vi "Initialize TreeBrowserWF.vi"(7 "guids":string[](array[string])=["4b95dee7-8d64-48ce-932c-f5fdd14e4d4c", "94e87467-031b-484c-a85e-bcbac581524d"], 8 "error in (no error)":errorcluster, 9 "Input Channels":cluster{"Node ID":u64}[](array[cluster]), 10 "Node Pointer":T1, 11 "TreeBrowserRef":refnum<k24>) -> (0 "error out":errorcluster, 2 "Channels":variant, 3 "TreeBrowserRef 2":refnum<k24>)   [LabVIEW 2023, in "Protection and Counter Support System Explorer.lvlib"]
uses:
  Protection and Counter Support System Explorer.lvlib
  <vilib>/NI VeriStand/Custom Device API/Custom Device Pointer.ctl
  NationalInstruments.VeriStand.SystemStorage
  NationalInstruments.VeriStand.SystemStorageUI
  NationalInstruments.VeriStand
  <vilib>/NI VeriStand/Custom Device API/Custom Device API.lvlib
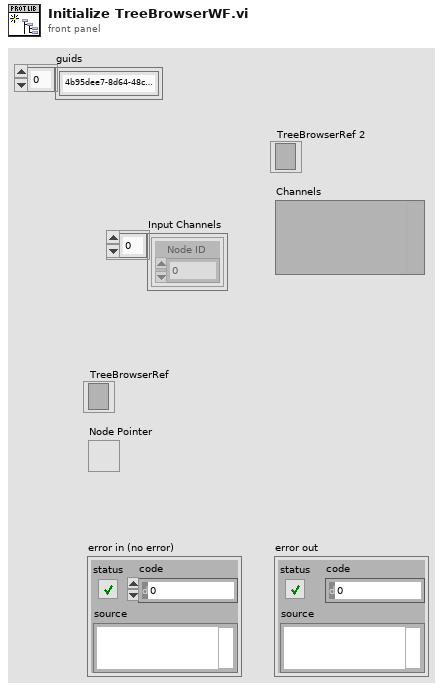
[diagram p1: front panel]
types:
  T1 = typedef "Custom Device API.lvlib/Custom Device Pointer.ctl" = refnum<k24>
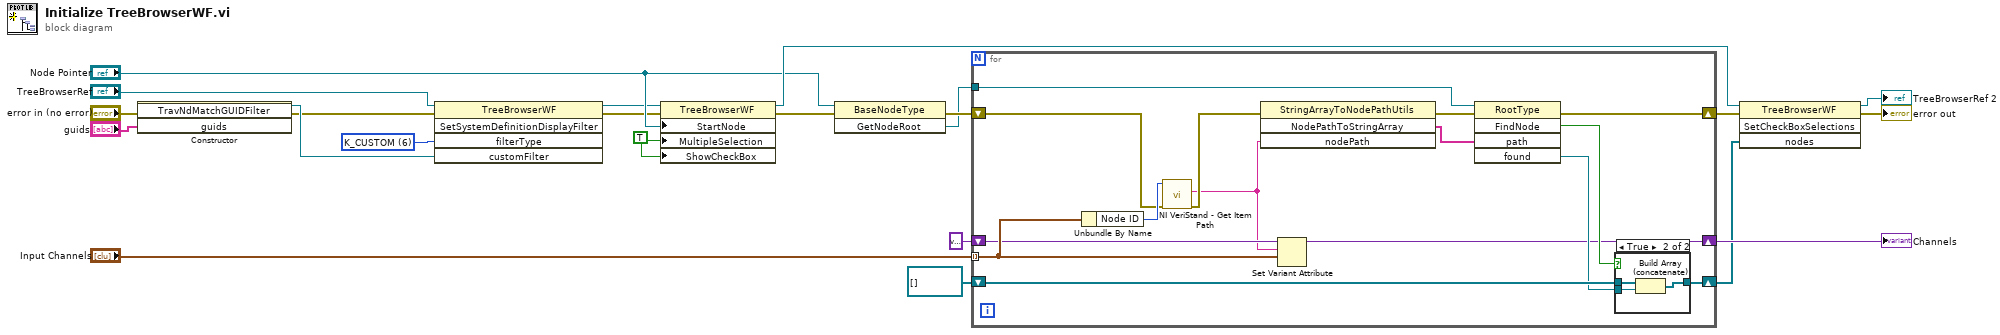
[diagram p0: block diagram]
diagram:
  w8 = u8 6 items=["K_CHAN_R", "K_CHAN_W", "K_CHAN_RW", "K_CHAN_VOLT", "K_CHAN_FAULT", "K_ALL", "K_CUSTOM", "K_CHAN_R_VIS", "K_CHAN_W_VIS", "K_CHAN_RW_VIS", "K_CHAN_VOLT_VIS", "K_CHAN_FAULT_VIS", "K_WAVE", "K_WAVE_VIS", "K_WAVE_DBL", "K_WAVE_CDB", "K_WAVE_DBL_VIS", "K_WAVE_CDB_VIS"] ("filterType")
  w17 = TRUE ("MultipleSelection")
  n1 = constructor class="TravNdMatchGUIDFilter"(error in="error in (no error)", "guids"="guids") -> (reference out=w6:refnum<k24>, error out=w5:errorcluster)  [unwired: 2 in, 2 out]
  n2 = invoke class="TreeBrowserWF" method="SetSystemDefinitionDisplayFilter"(reference="TreeBrowserRef", error in=w5, "filterType"=w8, "customFilter"=w6) -> (reference out=w2:refnum<k24>, error out=w4:errorcluster)  [unwired: 1 in, 3 out]
  n3 = property class="TreeBrowserWF"(reference=w2, error in=w4, "StartNode"="Node Pointer", "MultipleSelection"=w17, "ShowCheckBox"=w17) -> (reference out=w11:refnum<k24>, error out=w10:errorcluster)
  n4 = invoke class="BaseNodeType" method="GetNodeRoot"(reference="Node Pointer", error in=w10) -> (error out=w22:errorcluster, "GetNodeRoot"=w21:refnum<k24>)  [unwired: 1 in, 1 out]
  n5 = for {
    shift-right: [w34] -> w16
    shift-left: w22 -> [w25]
    tunnel: "Input Channels" -> [w29] mode=indexing
    tunnel: w21 -> [w37]
    shift-right: [w31] -> w18
    shift-left: refnum<k24>[] [] -> [w32]
    shift-right: [w27] -> w20
    shift-left: variant -> [w28]
    n6 = Unbundle By Name(w29) -> ("Node ID"=w26:u64)
    n7 = call <vilib>:"NI VeriStand - Get Item Path.vi"("error in (no error)"=w25, "Item Ref in"=w26) -> ("error out"=w24:errorcluster, "Path"=w23:string)  [unwired: 6 in, 2 out]
    n8 = invoke class="StringArrayToNodePathUtils" method="NodePathToStringArray"(error in=w24, "nodePath"=w23) -> (error out=w35:errorcluster, "NodePathToStringArray"=w36:string[])  [unwired: 2 in, 2 out]
    n9 = Set Variant Attribute(Variant=w28, name=w23, value=w29) -> (Variant out=w27:variant)  [unwired: 1 in, 2 out]
    n10 = invoke class="RootType" method="FindNode"(reference=w37, error in=w35, "path"=w36) -> (error out=w34:errorcluster, "FindNode"=w33:bool, "found"=w30:refnum<k24>)  [unwired: 2 in, 2 out]
    n11 = case shown="True" w33 {
      tunnel: w32 -> [w38 w41]
      tunnel: [w38 w39] -> w31
      tunnel: w30 -> [_ w40]
      frame False {
      }
      frame True {
        n12 = Build Array (concatenate)(w41, w40) -> (w39:refnum<k24>[])
      }
    }
  }
  "Channels" <- w20
  n13 = invoke class="TreeBrowserWF" method="SetCheckBoxSelections"(reference=w11, error in=w16, "nodes"=w18) -> (reference out=→"TreeBrowserRef 2":refnum<k24>, error out=→"error out":errorcluster)  [unwired: 1 in, 2 out]
